vi "calibrate_inv_kin.vi"(6 "Stimulus":sgl[][](array[numeric]), 7 "Decimated pose (manipulator)":dbl[][][](array[numeric]), 8 "Tip offset":sgl[](array[numeric])) -> (0 "Calibrated":T1, 1 "Error":dbl, 2 "New kinematics":T1 format="%#.3f", 3 "Handle coords output":dbl[][](array[numeric]) format="%#_3p")   [LabVIEW 2013]
uses:
  <vilib>/Analysis/Matrix/Datatypes/RealMatrix.ctl
  <vilib>/Analysis/baseanly.llb/A x Vector.vi
  <vilib>/Analysis/baseanly.llb/Real A x B.vi
  <vilib>/Analysis/_algsub.llb/Real PseudoInverse Matrix.vi
  <vilib>/Analysis/NI_AALPro.lvlib
  <vilib>/Analysis/NI_AALBase.lvlib
  <vilib>/Analysis/Matrix/NI_Matrix.lvlib
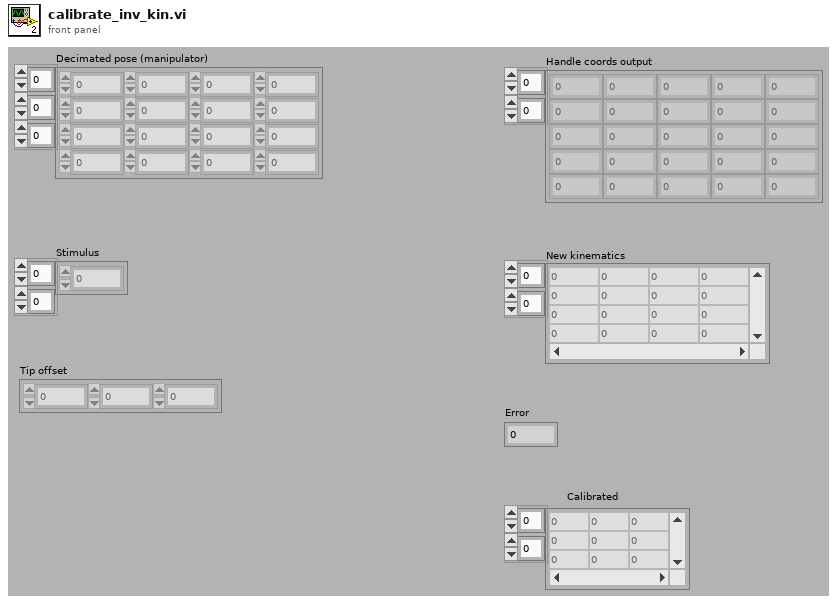
[diagram p1: front panel]
types:
  T1 = typedef "NI_Matrix.lvlib/RealMatrix.ctl" = dbl[][]
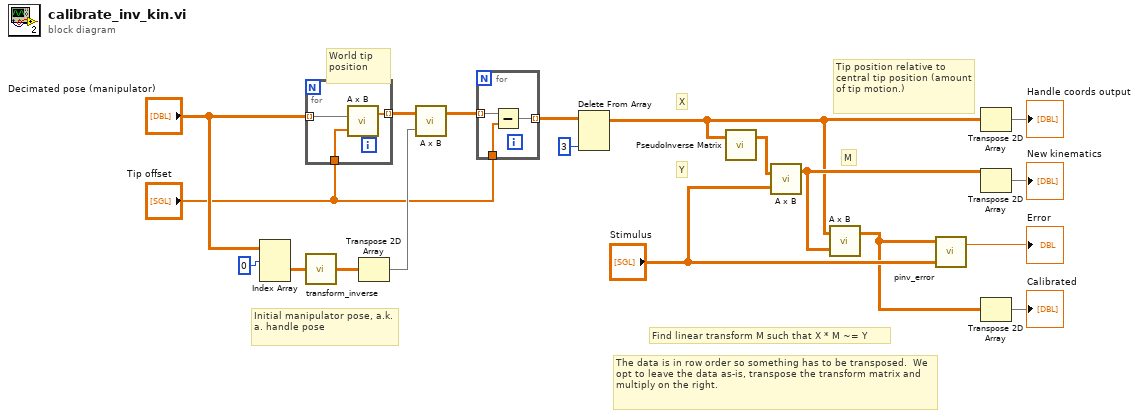
[diagram p0: block diagram]
diagram:
  # "The data is in row order so something has to be transposed.  We opt to leave the data as-is, transpose the transform matrix and multiply on the right."
  # "Tip position relative to central tip position (amount of tip motion.)"
  # "World tip position"
  # "Initial manipulator pose, a.k.a. handle pose"
  # "Find linear transform M such that X * M ~= Y"
  # "M"
  # "Y"
  # "X"
  n1 = Index Array(array="Decimated pose (manipulator)", index (dim 0)=0 ("index (page)")) -> (element=w10:dbl[][])  [unwired: 2 in]
  n2 = for {
    tunnel: "Decimated pose (manipulator)" -> [w21] mode=indexing
    tunnel: [w22] -> w7 mode=indexing
    tunnel: "Tip offset" -> [w20]
    n3 = call-poly <vilib>:"A x B.vi"("Vector"=w20, "A"=w21) -> ("A x Vector"=w22:dbl[])  [unwired: 1 out]
  }
  n4 = call "transform_inverse.vi"("Transform"=w10) -> ("Inverse transform"=w9:T1)
  n5 = Transpose 2D Array(2D array=w9) -> (transposed array=w8:T1)
  n6 = call-poly <vilib>:"A x B.vi"("B"=w8, "A"=w7) -> ("A x B"=w1:T1)  [unwired: 1 out]
  n7 = for {
    tunnel: w1 -> [w25] mode=indexing
    tunnel: "Tip offset" -> [w24]
    tunnel: [w23] -> w3 mode=indexing
    n8 = Subtract ("Subtract.vi")(x=w25, y=w24) -> (x-y=w23:dbl[])
  }
  n9 = Delete From Array(array=w3, index (col)=3 ("index (row)")) -> (array with subset deleted=w2:dbl[][])  [unwired: 2 in, 1 out]
  n10 = call-poly <vilib>:"PseudoInverse Matrix.vi"("Input Matrix"=w2) -> ("PseudoInverse Matrix"=w14:T1)  [unwired: 1 in, 1 out]
  n11 = call-poly <vilib>:"A x B.vi"("B"="Stimulus", "A"=w14) -> ("A x B"=w13:T1)  [unwired: 1 out]
  n12 = call-poly <vilib>:"A x B.vi"("B"=w13, "A"=w2) -> ("A x B"=w12:T1)  [unwired: 1 out]
  n13 = call "pinv_error.vi"("Y"="Stimulus", "Calibrated"=w12) -> ("Error"=→"Error":dbl)  [unwired: 1 in, 1 out]
  n14 = Transpose 2D Array(2D array=w2) -> (transposed array=→"Handle coords output":dbl[][])
  n15 = Transpose 2D Array(2D array=w13) -> (transposed array=→"New kinematics":T1)
  n16 = Transpose 2D Array(2D array=w12) -> (transposed array=→"Calibrated":T1)
